vi "Simulated VeriStand Engine.Interface.Allocate.Status Pointers.vi"(8 "error in (no error)":errorcluster, 11 "Simulated VeriStand Engine Interface in":refnum<class "Simulated VeriStand Engine.Interface.lvclass">) -> (0 "error out":errorcluster, 3 "Simulated VeriStand Engine Interface out":refnum<class "Simulated VeriStand Engine.Interface.lvclass">)   [LabVIEW 2016, in "Simulated VeriStand Engine.Interface.lvclass"]
uses:
  Simulated VeriStand Engine.Interface.lvclass
  Typedefs/Simulated VeriStand Engine.Interface.Pointers.Status.ctl
  Source/Submodules/Memory/Source/Classes/Internal/Memory.Pointer.Internal.lvclass
  Simulated VeriStand Engine.Interface.lvclass/Simulated VeriStand Engine.Interface.ctl
  Source/Submodules/Memory/Source/Classes/Internal/Memory.Pointer.Internal.Allocate.vi
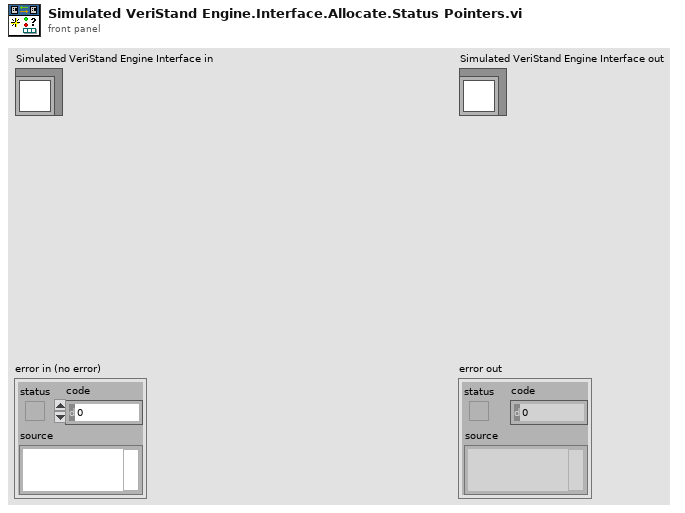
[diagram p1: front panel]
types:
  T1 = typedef "Simulated VeriStand Engine.Interface.lvclass/Simulated VeriStand Engine.Interface.Pointers.Status.ctl" = cluster{"Actual Period (µs)":refnum<class "Memory.Pointer.Internal.lvclass">}
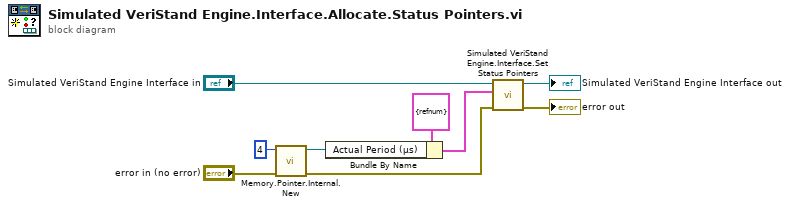
[diagram p0: block diagram]
diagram:
  n1 = call "Memory.Pointer.Internal.New.vi"("error in (no error)"="error in (no error)", "size"=u64 4) -> ("error out"=w3:errorcluster, "pointer"=w8:refnum<class "Memory.Pointer.Internal.lvclass">)  [unwired: 8 in]
  n2 = Bundle By Name(cluster=T1 {"Actual Period (µs)"=refnum} ("Status Pointers"), "Actual Period (µs)"=w8) -> (w2:T1)
  n3 = call "Simulated VeriStand Engine.Interface.Set Status Pointers.vi"("error in (no error)"=w3, "Status Pointers"=w2, "Simulated VeriStand Engine Interface in"="Simulated VeriStand Engine Interface in") -> ("error out"=→"error out":errorcluster, "Simulated VeriStand Engine Interface out"=→"Simulated VeriStand Engine Interface out":refnum<class "Simulated VeriStand Engine.Interface.lvclass">)  [unwired: 7 in]
